vi "Untitled 4.vi"() -> ()   [LabVIEW 2019]
uses:
  <vilib>/Platform/TimedLoop/XDataNode/timing_clust.ctl
  <vilib>/Platform/TimedLoop/XDataNode/nitl_modes.ctl
  <vilib>/Platform/TimedLoop/XDataNode/wakeup.ctl
  <vilib>/imath/engines/lvmath2/RunTimeEngine/BuiltInFunctions/diag/NIMS_diag.vi
  <instcachedir>/0/NIMS_diag_DCAB8C8FDAF64F9E84492BB524435AA9.lvgen/NIMS_diag_DCAB8C8FDAF64F9E84492BB524435AA9_003.vi
  <vilib>/imath/engines/lvmath2/RunTimeEngine/RowToken/NIMS_RowToken_M_M.vi
  <instcachedir>/0/NIMS_RowToken_M_M_21FE36D058524603B8B587AC30FD72C2.lvgen/NIMS_RowToken_M_M_21FE36D058524603B8B587AC30FD72C2_005.vi
  <vilib>/imath/engines/lvmath2/RunTimeEngine/BuiltInFunctions/mirrorh/NIMS_mirrorh(GM).vi
  <instcachedir>/0/NIMS_mirrorh(GM)_A650AD0D730A4A8EBE251B4C5C7CA115.lvgen/NIMS_mirrorh(GM)_A650AD0D730A4A8EBE251B4C5C7CA115_004.vi
  <vilib>/imath/engines/lvmath2/RunTimeEngine/ErrorHandling/NIMS_Create Error From Enums.vi
  <vilib>/imath/engines/lvmath2/RunTimeEngine/NodeEndStatement/NIMS_NodeEndStatement_Output.vi
  <instcachedir>/0/NIMS_NodeEndStatement_Output_53EC0D466D134D7ABD903AC30B43404B.lvgen/NIMS_NodeEndStatement_Output_53EC0D466D134D7ABD903AC30B43404B_005.vi
  <instcachedir>/0/NIMS_NodeEndStatement_Output_53EC0D466D134D7ABD903AC30B43404B.lvgen/NIMS_NodeEndStatement_Output_53EC0D466D134D7ABD903AC30B43404B_002.vi
  <instcachedir>/0/NIMS_NodeEndStatement_Output_53EC0D466D134D7ABD903AC30B43404B.lvgen/NIMS_NodeEndStatement_Output_53EC0D466D134D7ABD903AC30B43404B_010.vi
  <vilib>/imath/engines/lvmath2/RunTimeEngine/ErrorHandling/NIMS_Finalize Error.vi
  <vilib>/imath/engines/lvmath2/RunTimeEngine/BuiltInFunctions/length/NIMS_length(GV).vi
  <instcachedir>/0/NIMS_length(GV)_08A3D13377FD4E4B96F5795FBF3698FA.lvgen/NIMS_length(GV)_08A3D13377FD4E4B96F5795FBF3698FA_000.vi
  LabVIEW Data/MathScriptVIs/MCStatic_41946317732_5a8e250eb30f34e82135cccebbd5303c.vi
  <instcachedir>/0/MCStatic_41946317732_5a8e250eb30f34e82135cccebbd5303c_B084D7F86B0340018A816984B2AA8430.lvgen/MCStatic_41946317732_5a8e250eb30f34e82135cccebbd5303c_B084D7F86B0340018A816984B2AA8430_001.vi
  <vilib>/imath/engines/lvmath2/RunTimeEngine/ArithmeticOperatorToken/NIMS_ArithmeticOperator_multmx.vi
  <instcachedir>/0/NIMS_ArithmeticOperator_multmx_77F1D2D6F4D94BA7A97C4E7185C02392.lvgen/NIMS_ArithmeticOperator_multmx_77F1D2D6F4D94BA7A97C4E7185C02392_003.vi
  <instcachedir>/0/NIMS_diag_DCAB8C8FDAF64F9E84492BB524435AA9.lvgen/NIMS_diag_DCAB8C8FDAF64F9E84492BB524435AA9_002.vi
  <vilib>/imath/engines/lvmath2/RunTimeEngine/BuiltInFunctions/max/1 input/NIMS_max(CM).vi
  <instcachedir>/0/NIMS_max(CM)_ECFF9CEF2CF74B92B05BC258ECD38873.lvgen/NIMS_max(CM)_ECFF9CEF2CF74B92B05BC258ECD38873_000.vi
  <vilib>/imathl/engines/lvmath/Functions/Error Handling/Create Error.vi
  <vilib>/imath/engines/lvmath/Functions/Error Handling/MergeErrorsWrapper.vi
  <vilib>/imath/engines/lvmath2/RunTimeEngine/CommandStatement/MC_CommandStatement_break.vi
  LabVIEW Data/MathScriptVIs/MCStatic_41946317732_dd0a4abc983190fa8a6f1d8969b5664d.vi
  <instcachedir>/0/MCStatic_41946317732_dd0a4abc983190fa8a6f1d8969b5664d_8BF022BAB4A64A2E8D63348063E331ED.lvgen/MCStatic_41946317732_dd0a4abc983190fa8a6f1d8969b5664d_8BF022BAB4A64A2E8D63348063E331ED_000.vi
  <vilib>/imath/engines/lvmath2/RunTimeEngine/ArithmeticOperatorToken/NIMS_ArithmeticOperator_minus.vi
  <instcachedir>/0/NIMS_ArithmeticOperator_minus_12BFF9710EA5430A9EE87C5BC3F65186.lvgen/NIMS_ArithmeticOperator_minus_12BFF9710EA5430A9EE87C5BC3F65186_009.vi
  <vilib>/imath/engines/lvmath2/RunTimeEngine/BuiltInFunctions/norm/NIMS_norm(GM,DBL).vi
  <instcachedir>/0/NIMS_norm(GM,DBL)_8BCB088F207E48DF95CF5C1DC502F84D.lvgen/NIMS_norm(GM,DBL)_8BCB088F207E48DF95CF5C1DC502F84D_001.vi
  <vilib>/imath/engines/lvmath2/RunTimeEngine/BuiltInFunctions/abs/NIMS_abs(signed).vi
  <instcachedir>/0/NIMS_abs(signed)_C4FCB8E6058B49B797C7C8D53CA5F6EC.lvgen/NIMS_abs(signed)_C4FCB8E6058B49B797C7C8D53CA5F6EC_003.vi
  <vilib>/imath/engines/lvmath2/RunTimeEngine/BuiltInFunctions/max/1 input/NIMS_max(RM).vi
  <instcachedir>/0/NIMS_max(RM)_0B4294876EE440609D638D7C5C6E788E.lvgen/NIMS_max(RM)_0B4294876EE440609D638D7C5C6E788E_000.vi
  <vilib>/imath/engines/lvmath2/RunTimeSupport/NIMS_Get Scalar_w Error.vi
  <instcachedir>/0/NIMS_Get Scalar_w Error_90FA09EFB1C84794B43793796939E0E3.lvgen/NIMS_Get Scalar_w Error_90FA09EFB1C84794B43793796939E0E3_010.vi
  <vilib>/imath/engines/lvmath2/RunTimeEngine/BuiltInFunctions/eye/NIMS_M=eye(I32).vi
  <instcachedir>/0/NIMS_ArithmeticOperator_multmx_77F1D2D6F4D94BA7A97C4E7185C02392.lvgen/NIMS_ArithmeticOperator_multmx_77F1D2D6F4D94BA7A97C4E7185C02392_006.vi
  <vilib>/imath/engines/lvmath2/RunTimeEngine/ArithmeticOperatorToken/NIMS_ArithmeticOperator_plus.vi
  <instcachedir>/0/NIMS_ArithmeticOperator_plus_5C9385B0197D46E2B844C41E02F9EC39.lvgen/NIMS_ArithmeticOperator_plus_5C9385B0197D46E2B844C41E02F9EC39_002.vi
  <vilib>/imath/engines/lvmath2/RunTimeEngine/ArithmeticOperatorToken/NIMS_ArithmeticOperator_leftdivmx(C,C).vi
  <instcachedir>/0/NIMS_ArithmeticOperator_leftdivmx(C,C)_FFA86DC98B994D28AA7593516F1DAFDA.lvgen/NIMS_ArithmeticOperator_leftdivmx(C,C)_FFA86DC98B994D28AA7593516F1DAFDA_000.vi
  <vilib>/imath/engines/lvmath2/RunTimeEngine/ArithmeticOperatorToken/NIMS_ArithmeticOperator_rightdiv.vi
  <instcachedir>/0/NIMS_ArithmeticOperator_rightdiv_23AAA10E4B1E4564B1AF1956090A34B0.lvgen/NIMS_ArithmeticOperator_rightdiv_23AAA10E4B1E4564B1AF1956090A34B0_004.vi
  <vilib>/imath/engines/lvmath2/RunTimeEngine/BuiltInFunctions/is_finite/NIMS_is_finite.vi
  <instcachedir>/0/NIMS_is_finite_E890EE136B8C42F1894B8FB6CFD6E9D7.lvgen/NIMS_is_finite_E890EE136B8C42F1894B8FB6CFD6E9D7_001.vi
  <vilib>/imath/engines/lvmath2/RunTimeEngine/BuiltInFunctions/all/NIMS_all(GM).vi
  <instcachedir>/0/NIMS_ArithmeticOperator_minus_12BFF9710EA5430A9EE87C5BC3F65186.lvgen/NIMS_ArithmeticOperator_minus_12BFF9710EA5430A9EE87C5BC3F65186_008.vi
  <vilib>/imath/engines/lvmath2/RunTimeEngine/ArithmeticOperatorToken/NIMS_ArithmeticOperator_rightdivmx(C,C).vi
  <instcachedir>/0/NIMS_ArithmeticOperator_rightdivmx(C,C)_4C9834AF73264B85B2EC0ABB36B07CCF.lvgen/NIMS_ArithmeticOperator_rightdivmx(C,C)_4C9834AF73264B85B2EC0ABB36B07CCF_000.vi
  <vilib>/imath/engines/lvmath2/RunTimeEngine/ArithmeticOperatorToken/NIMS_ArithmeticOperator_powermx(M,M).vi
  <vilib>/imath/engines/lvmath2/RunTimeEngine/BuiltInFunctions/max/2 inputs/NIMS_max(CG,CG)-no size check.vi
  <instcachedir>/0/NIMS_max(CG,CG)-no size check_0D8807EB624448B1961BA94FD6C7666D.lvgen/NIMS_max(CG,CG)-no size check_0D8807EB624448B1961BA94FD6C7666D_000.vi
  <instcachedir>/0/MCStatic_41946317732_5a8e250eb30f34e82135cccebbd5303c_B084D7F86B0340018A816984B2AA8430.lvgen/MCStatic_41946317732_5a8e250eb30f34e82135cccebbd5303c_B084D7F86B0340018A816984B2AA8430_000.vi
  <vilib>/imath/engines/lvmath2/RunTimeEngine/CommandStatement/NIMS_CommandStatement_MaskErr.vi
  <vilib>/platform/TimedLoop/XDataNode/XDataNode.xnode
  Analytic_Jacobian_Mag_cir_array_test.m
  PM_forward_field.m
  <vilib>/Platform/TimedLoop/XDataNode/XDNodeRunTimeDep.lvlib
  <instcachedir>/0/MCStatic_41946317732_dd0a4abc983190fa8a6f1d8969b5664d_8BF022BAB4A64A2E8D63348063E331ED.lvgen/MCStatic_41946317732_dd0a4abc983190fa8a6f1d8969b5664d_8BF022BAB4A64A2E8D63348063E331ED_001.vi
panel:
  out "pm_hat_opt":dbl[][](array[numeric])
  out "Late cycles":u16
  in  "stop":bool
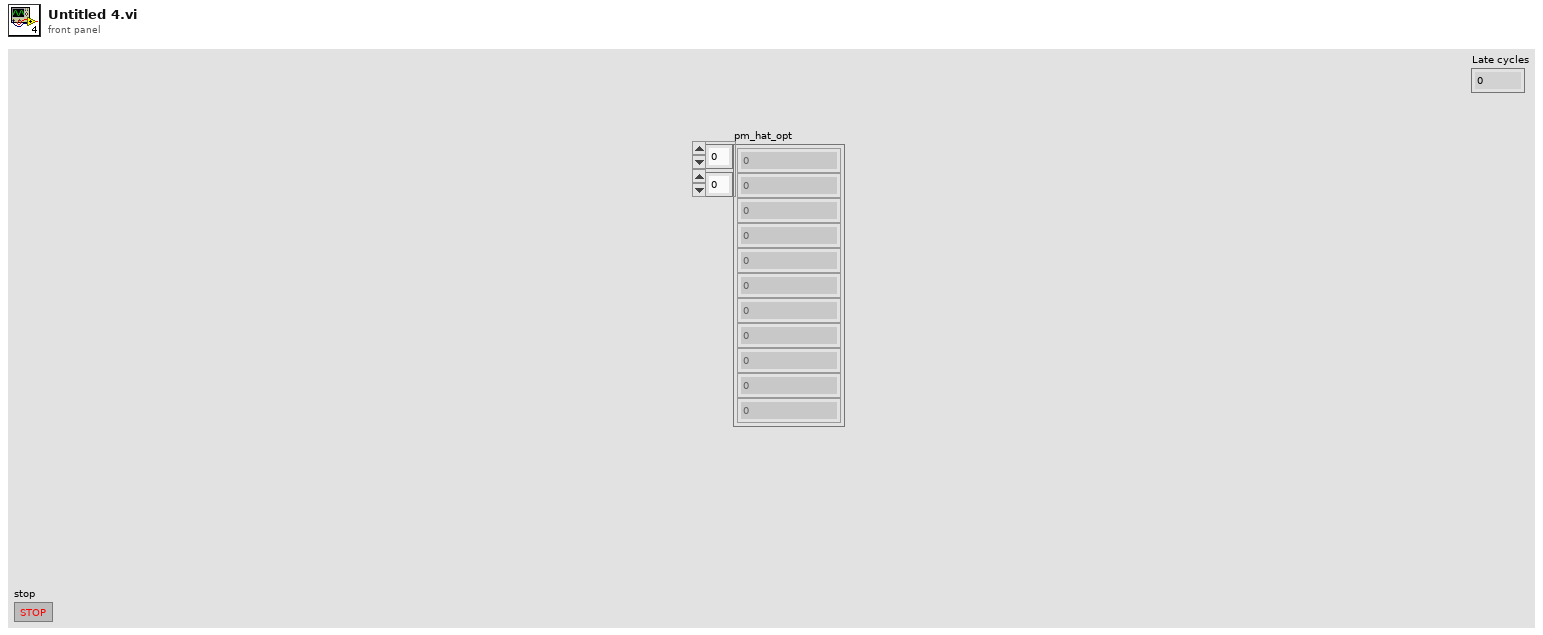
[diagram p1: front panel]
types:
  T1 = typedef "XDNodeRunTimeDep.lvlib/timing_clust.ctl" = cluster{"Expected End [f-1]":u64, "Actual End [f-1]":u64, "Finished Late? [f-1]":bool, "Expected End [i-1]":u64, "Actual End [i-1]":u64, "Finished Late? [i-1]":bool, "Expected Start [i]":u64, "Actual Start [i]":u64, "Expected Start [f]":u64, "Actual Start [f]":u64, "Source Name":string, "Structure Name":string, "Period":i64, "Deadline":i64, "Offset":i64, "Start":i64, "Priority":i32, "Timeout":i32, "Mode":T2, "Wakeup Reason":T3, "Error":errorcluster, "Source Type":string, "Secondary Source Type":string, "Global End Time":u64, "Global Start Time":u64, "Frame Duration":u64, "Iteration Duration":u64, "Assigned CPU":i32, "I/O Scan Engine Mode":u32}
  T2 = typedef "XDNodeRunTimeDep.lvlib/nitl_modes.ctl" = enum32{"No Change", "Process missed periods, maintain original phase", "Discard missed periods, maintain original phase", "Process missed periods, ignore original phase", "Discard missed periods, ignore original phase"}
  T3 = typedef "XDNodeRunTimeDep.lvlib/wakeup.ctl" = enum32{"Normal", "Aborted", "Asynchronous wakeup", "Timing source error", "Timed loop error", "Timeout"}
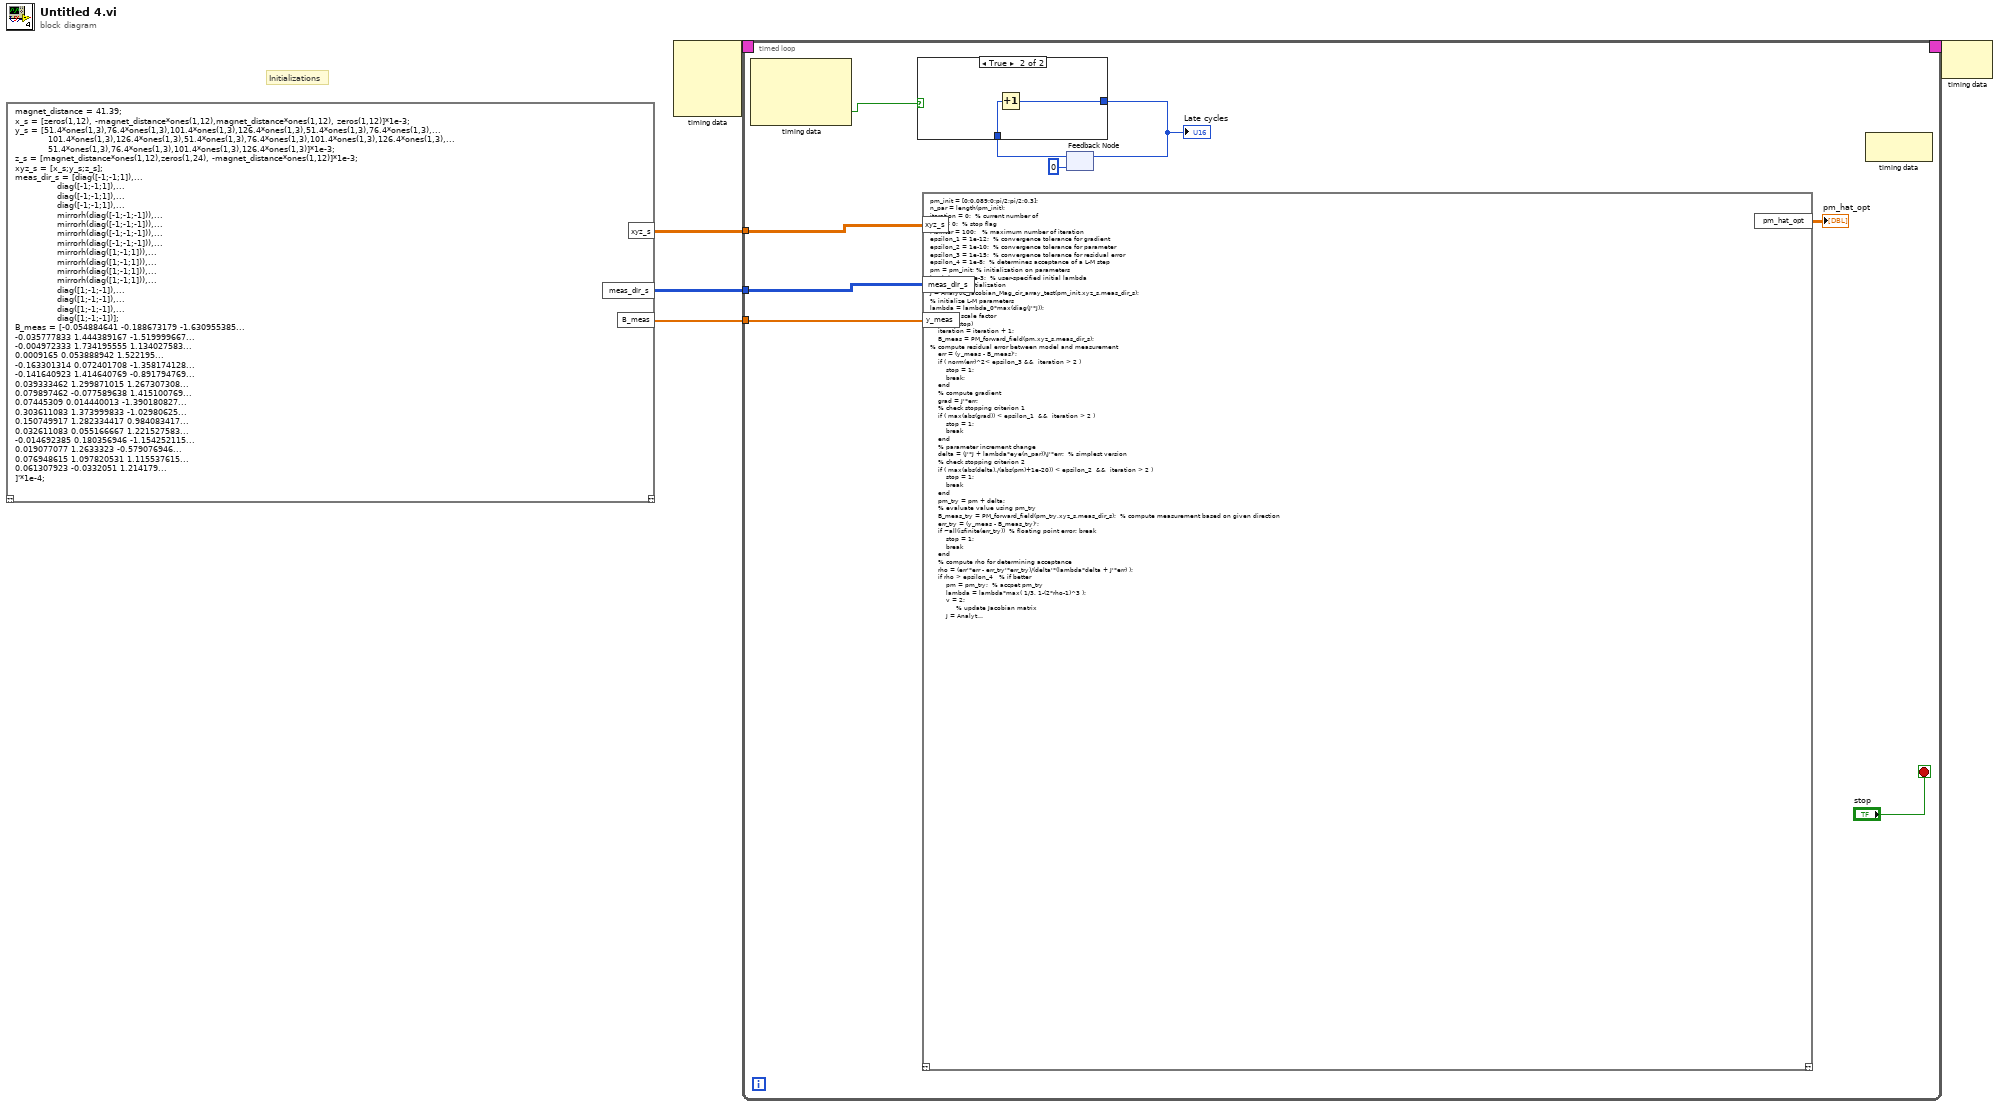
[diagram p0: block diagram]
diagram:
  # "Initializations"
  n1 = mathscript code="magnet_distance = 41.39;\nx_s = [zeros(1,12), -magnet_distance*ones(1,12),magnet_distance*ones(1,12), zeros(1,12)]*1e-3; \ny_s = [51.4*ones(1,3),76.4*ones(1,3),101.4*ones(1,3),126.4*ones(1,3),51.4*ones(1,3),76.4*ones(1,3),...\n           101.4*ones(1,3),126.4*ones(1,3),51.4*ones(1,3),76.4*ones(1,3),101.4*ones(1,3),126.4*ones(1,3),...\n           51.4*ones(1,3),76.4*ones(1,3),101.4*ones(1,3),126.4*ones(1,3)]*1e-3; \nz_s = [magnet_distance*ones(1,12),zeros(1,24), -magnet_distance*ones(1,12)]*1e-3; \nxyz_s = [x_s;y_s;z_s];  \nmeas_dir_s = [diag([-1;-1;1]),...\n              diag([-1;-1;1]),...\n              diag([-1;-1;1]),...\n              diag([-1;-1;1]),...\n              mirrorh(diag([-1;-1;-1])),...\n              mirrorh(diag([-1;-1;-1])),...\n              mirrorh(diag([-1;-1;-1])),...\n              mirrorh(diag([-1;-1;-1])),...\n              mirrorh(diag([1;-1;1])),...\n              mirrorh(diag([1;-1;1])),...\n              mirrorh(diag([1;-1;1])),...\n              mirrorh(diag([1;-1;1])),...\n              diag([1;-1;-1]),...\n              diag([1;-1;-1]),...\n              diag([1;-1;-1]),...\n              diag([1;-1;-1])];\nB_meas = [-0.054884641\t-0.188673179\t-1.630955385...\n-0.035777833\t1.444389167\t-1.519999667...\n-0.004972333\t1.734195555\t1.134027583...\n0.0009165\t0.053888942\t1.522195...\n-0.163301314\t0.072401708\t-1.358174128...\n-0.141640923\t1.414640769\t-0.891794769...\n0.039333462\t1.299871015\t1.267307308...\n0.079897462\t-0.077589638\t1.415100769...\n0.07445309\t0.014440013\t-1.390180827...\n0.303611083\t1.373999833\t-1.02980625...\n0.150749917\t1.282334417\t0.984083417...\n0.032611083\t0.055166667\t1.221527583...\n-0.014692385\t0.180356946\t-1.154252115...\n0.019077077\t1.2633323\t-0.579076946...\n0.076948615\t1.097820531\t1.115537615...\n0.061307923\t-0.0332051\t1.214179...\n]'*1e-4;"() -> ("meas_dir_s"=w3:i32[][], "xyz_s"=w2:dbl[][], "B_meas"=w1:dbl[])  [unwired: 1 in, 1 out]
  n2 = node-c288() -> (w5:T1)  [unwired: 4 in]
  n3 = timed-loop {
    timing: w5 -> [_]
    timing-out: [_] -> w4
    tunnel: w3 -> [w13]
    tunnel: w2 -> [w12]
    tunnel: w1 -> [w7]
    stop <- "stop" stop-if-true
    n4 = node-c288() -> (w11:bool)  [unwired: 1 in, 3 out]
    n5 = mathscript code="pm_init = [0;0.089;0;pi/2;pi/2;0.3];\nn_par = length(pm_init);\niteration = 0;  % current number of \nstop = 0;  % stop flag\nMaxIter = 100;   % maximum number of iteration\nepsilon_1 = 1e-12;  % convergence tolerance for gradient\nepsilon_2 = 1e-10;  % convergence tolerance for parameter\nepsilon_3 = 1e-15;  % convergence tolerance for residual error\nepsilon_4 = 1e-8;  % determines acceptance of a L-M step\npm = pm_init; % initialization on parameters\nlambda_0 = 1e-3;  % user-specified initial lambda\n% Jacobian initialization\nJ = Analytic_Jacobian_Mag_cir_array_test(pm_init,xyz_s,meas_dir_s);\n% initialize L-M parameters\nlambda = lambda_0*max(diag(J'*J));\nv = 2;  % scale factor\nwhile ( ~stop)\n    iteration = iteration + 1;\n    B_meas = PM_forward_field(pm,xyz_s,meas_dir_s);\n% compute residual error between model and measurement\n    err = (y_meas - B_meas)';\n    if ( norm(err)^2< epsilon_3 &&  iteration > 2 )\n        stop = 1;\n        break;\n    end\n    % compute gradient\n    grad = J'*err;\n    % check stopping criterion 1\n    if ( max(abs(grad)) < epsilon_1  &&  iteration > 2 )\n        stop = 1;\n        break\n    end\n    % parameter increment change\n    delta = (J'*J + lambda*eye(n_par))\\J'*err;  % simplest version\n    % check stopping criterion 2 \n    if ( max(abs(delta)./(abs(pm)+1e-20)) < epsilon_2  &&  iteration > 2 )\n        stop = 1;\n        break\n    end\n    pm_try = pm + delta;\n    % evaluate value using pm_try\n    B_meas_try = PM_forward_field(pm_try,xyz_s,meas_dir_s);  % compute measurement based on given direction\n    err_try = (y_meas - B_meas_try)';\n    if ~all(isfinite(err_try))  % floating point error; break\n        stop = 1;\n        break\n    end\n    % compute rho for determining acceptance\n    rho = (err'*err - err_try'*err_try)/(delta'*(lambda*delta + J'*err) );\n    if rho > epsilon_4   % if better\n        pm = pm_try;  % accpet pm_try\n        lambda = lambda*max( 1/3, 1-(2*rho-1)^3 );\n        v = 2;\n             % update Jacobian matrix\n        J = Analytic_Jacobian_Mag_cir_array_test(pm,xyz_s,meas_dir_s);\n    else      % if not better\n        lambda = lambda*v;\n        v = 2*v;\n    end\n    if ( iteration == MaxIter )\n        stop = 1;\n    end\nend\n\npm_hat_opt = pm;"("meas_dir_s"=w13, "xyz_s"=w12, "y_meas"=w7) -> ("pm_hat_opt"=→"pm_hat_opt":dbl[][])  [unwired: 1 in, 1 out]
    n6 = feedback #1(u16 0) -> (w10:u16)
    n7 = case shown="True" w11 {
      tunnel: w10 -> [w15 w17]
      tunnel: [w15 w16] -> w9
      frame False {
      }
      frame True {
        n8 = Increment(x=w17) -> (x+1=w16:u16)
      }
    }
    "Late cycles" <- w9
    n9 = feedback-in #1(w9) -> ()
    n10 = node-c288() -> ()  [unwired: 1 in, 1 out]
  }
  n11 = node-c288(w4) -> ()  [unwired: 1 out]
